vi "realtime_I_K6221_vs_time_PK.vi"() -> ()   [LabVIEW 2016]
uses:
  <instrlib>/Keithley 622x LV 2009/Utility/Typedefs/KE622x -- Instrument Type.ctl
  <instrlib>/Keithley 622x LV 2009/Keithley 622x.lvlib
panel:
  in  "Instrument Type":T1=enum."KE6221"
  in  "K6221":refnum<visa-resource-name>="GPIB0::26::INSTR"
  out "Time(s)":dbl format="%#_13g"
  out "No. of data points collected":i32
  out "Current (A)":dbl=nan
  out "Current vs time":cluster{dbl, "Field Reading":dbl}[](graph)=[{0.0, "Field Reading"=1.0754909033057532e-08}, {4.551, "Field Reading"=1.0775176727399796e-08}, {9.079, "Field Reading"=1.0695936548822218e-08}, {13.636, "Field Reading"=1.0701268908690468e-08}, {18.154, "Field Reading"=1.0658796866433243e-08}, {22.685, "Field Reading"=1.0644955615895597e-08}, {27.196, "Field Reading"=1.0609443608454975e-08}, {31.764, "Field Reading"=1.0588135917913612e-08}, {36.283, "Field Reading"=1.0537267739517534e-08}, {40.802, "Field Reading"=1.0571090092717568e-08}, {45.37, "Field Reading"=1.0597450432074013e-08}, {49.892, "Field Reading"=1.0554082828015275e-08}, {54.416, "Field Reading"=1.0529144396930967e-08}, {58.975, "Field Reading"=1.0525243011530484e-08}, {63.495, "Field Reading"=1.0496422204909802e-08}, {68.076, "Field Reading"=1.0537492386015997e-08}, {72.594, "Field Reading"=1.041855360011532e-08}, {77.111, "Field Reading"=1.0414805764361074e-08}, {81.633, "Field Reading"=1.0427666088764133e-08}, {86.192, "Field Reading"=1.040983248991928e-08}, {90.711, "Field Reading"=1.0415274184948404e-08}, {95.278, "Field Reading"=1.0351658780517077e-08}, {99.809, "Field Reading"=1.0347778042711309e-08}, {104.32, "Field Reading"=1.0404151525170418e-08}, {108.897, "Field Reading"=1.0367328564547418e-08}, {113.406, "Field Reading"=1.035592250362828e-08}, {117.929, "Field Reading"=1.034164711520283e-08}, {122.501, "Field Reading"=1.0372545079311634e-08}, {127.022, "Field Reading"=1.035853398570497e-08}, {131.534, "Field Reading"=1.0266362316389294e-08}, {136.112, "Field Reading"=1.0243831678579991e-08}, {140.623, "Field Reading"=1.0293090037428198e-08}, {145.201, "Field Reading"=1.025001076059906e-08}, {149.713, "Field Reading"=1.0220389068636026e-08}, {154.229, "Field Reading"=1.0367862293665633e-08}, {158.755, "Field Reading"=1.0208599005305017e-08}, {163.317, "Field Reading"=1.0248389252815388e-08}, {167.846, "Field Reading"=1.0199880715923942e-08}, {172.357, "Field Reading"=1.020809912913377e-08}, {176.927, "Field Reading"=1.0004231807512444e-08}, {181.447, "Field Reading"=1.0056198083741343e-08}, {186.01, "Field Reading"=1.0175625482064012e-08}, {190.532, "Field Reading"=1.01869251911497e-08}, {195.05, "Field Reading"=1.0021725360158898e-08}, {199.622, "Field Reading"=1.0012994392348114e-08}, {204.146, "Field Reading"=9.997701041555824e-09}, {208.72, "Field Reading"=1.0014654313310312e-08}, {213.225, "Field Reading"=1.0025557506602398e-08}, {217.746, "Field Reading"=1.0035240153436886e-08}, {222.264, "Field Reading"=9.984295354303873e-09}, {226.836, "Field Reading"=9.945901881505377e-09}, {231.363, "Field Reading"=9.909901055069444e-09}, {235.87, "Field Reading"=9.879079688367416e-09}, {240.45, "Field Reading"=9.871891153879234e-09}, {244.957, "Field Reading"=9.820091191293928e-09}, {249.483, "Field Reading"=9.868208637490788e-09}, {254.057, "Field Reading"=9.723922102520499e-09}, {258.569, "Field Reading"=9.810851178546986e-09}, {263.137, "Field Reading"=9.868075070608025e-09}, {267.653, "Field Reading"=9.838459710300165e-09}, {272.232, "Field Reading"=9.794170154639246e-09}, {276.743, "Field Reading"=9.8240656612309e-09}, {281.263, "Field Reading"=9.816160129037189e-09}, {285.784, "Field Reading"=9.76028149014062e-09}, {290.358, "Field Reading"=9.770277657564933e-09}, {294.874, "Field Reading"=9.746852359819687e-09}, {299.449, "Field Reading"=9.691761324726048e-09}, {303.963, "Field Reading"=9.684356029780129e-09}, {308.532, "Field Reading"=9.679807729280934e-09}, {313.057, "Field Reading"=9.640167724579342e-09}, {317.576, "Field Reading"=9.651175663070228e-09}, {322.083, "Field Reading"=9.58822823601118e-09}, {326.663, "Field Reading"=9.599135974960226e-09}, {331.185, "Field Reading"=9.598302330065866e-09}, {335.749, "Field Reading"=9.594917386794453e-09}, {340.262, "Field Reading"=9.525752610701409e-09}, {344.782, "Field Reading"=9.535515829352e-09}, {349.309, "Field Reading"=9.561137526842156e-09}, {353.874, "Field Reading"=9.584085744924857e-09}, {358.396, "Field Reading"=9.477114337135297e-09}, {362.912, "Field Reading"=9.447686796961366e-09}, {367.477, "Field Reading"=9.456034130056011e-09}, {372.052, "Field Reading"=9.553141057667689e-09}, {376.566, "Field Reading"=9.493894961055902e-09}, {381.085, "Field Reading"=9.512667690597965e-09}, {385.602, "Field Reading"=9.474293153796591e-09}, {390.171, "Field Reading"=9.48223505565176e-09}, {394.688, "Field Reading"=9.445833232680502e-09}, {399.211, "Field Reading"=9.435606847282211e-09}, {403.78, "Field Reading"=9.392508049903565e-09}, {408.307, "Field Reading"=9.449390881958631e-09}, {412.825, "Field Reading"=9.387147868215114e-09}, {417.398, "Field Reading"=9.385493712017552e-09}, {421.906, "Field Reading"=9.400358378971229e-09}, {426.424, "Field Reading"=9.398262149895849e-09}, {430.944, "Field Reading"=9.293325719135014e-09}, {435.509, "Field Reading"=9.25682735507907e-09}, {440.034, "Field Reading"=9.374365520285052e-09}, {444.553, "Field Reading"=9.318008914318868e-09}, {449.118, "Field Reading"=9.379955683639186e-09}, {453.644, "Field Reading"=9.253105241135013e-09}, {458.209, "Field Reading"=9.328575358279307e-09}, {462.734, "Field Reading"=9.253544243941528e-09}, {467.255, "Field Reading"=9.25991158545122e-09}, {471.816, "Field Reading"=9.284130103339946e-09}, {476.34, "Field Reading"=9.260943222993443e-09}, {480.855, "Field Reading"=9.221960949633347e-09}, {485.445, "Field Reading"=9.185801120431644e-09}, {489.94, "Field Reading"=9.159181944365167e-09}, {494.463, "Field Reading"=9.209935281527626e-09}, {499.034, "Field Reading"=9.19608375149852e-09}, {503.556, "Field Reading"=9.182985788676442e-09}, {508.068, "Field Reading"=9.165322100062373e-09}, {512.638, "Field Reading"=9.211178101816789e-09}, {517.158, "Field Reading"=9.180204858998693e-09}, {521.685, "Field Reading"=9.158994559236158e-09}, {526.255, "Field Reading"=9.1758963250259e-09}, {530.765, "Field Reading"=9.086634986873923e-09}, {535.28, "Field Reading"=9.099900873430183e-09}, {539.853, "Field Reading"=9.120829376096234e-09}, {544.369, "Field Reading"=9.087269332815875e-09}, {548.898, "Field Reading"=9.082007695288655e-09}, {553.458, "Field Reading"=9.214812031637344e-09}, {557.978, "Field Reading"=9.11252387708823e-09}, {562.496, "Field Reading"=9.072929736222325e-09}, {567.068, "Field Reading"=9.021043183178307e-09}, {571.584, "Field Reading"=9.03801125958304e-09}, {576.105, "Field Reading"=9.01631848737752e-09}, {580.673, "Field Reading"=9.050041364125796e-09}, {585.2, "Field Reading"=8.977713001804232e-09}, {589.721, "Field Reading"=8.99190890091733e-09}, {594.28, "Field Reading"=8.971478919836577e-09}, {598.808, "Field Reading"=9.086145460689195e-09}, {603.368, "Field Reading"=9.02352800831983e-09}, {607.894, "Field Reading"=9.006141316948349e-09}, {612.406, "Field Reading"=8.971321772943122e-09}, {616.977, "Field Reading"=8.87637227658503e-09}, {621.495, "Field Reading"=8.996522434369188e-09}, {626.065, "Field Reading"=8.950902247062842e-09}, {630.587, "Field Reading"=8.912383643615826e-09}, {635.103, "Field Reading"=8.976870354539083e-09}, {639.673, "Field Reading"=8.858923858160401e-09}, {644.201, "Field Reading"=8.8960051768792e-09}, {648.72, "Field Reading"=8.810199581584296e-09}, {653.288, "Field Reading"=8.895940941745202e-09}, {657.806, "Field Reading"=8.899913022850807e-09}, {662.319, "Field Reading"=8.916190881138338e-09}, {666.887, "Field Reading"=8.924042487696841e-09}, {671.406, "Field Reading"=8.914859635649715e-09}, {675.933, "Field Reading"=8.853835406217462e-09}, {680.445, "Field Reading"=8.878049398532991e-09}, {684.96, "Field Reading"=8.838628299924819e-09}, {689.49, "Field Reading"=8.86209668870415e-09}, {694.002, "Field Reading"=8.995111648514265e-09}, {698.574, "Field Reading"=8.83478014979106e-09}, {703.094, "Field Reading"=8.717619560190315e-09}, {707.609, "Field Reading"=8.712050013497354e-09}, {712.124, "Field Reading"=8.708502365357036e-09}, {716.696, "Field Reading"=8.691314966662255e-09}, {721.217, "Field Reading"=8.737746080764506e-09}, {725.797, "Field Reading"=8.754542348338075e-09}, {730.303, "Field Reading"=8.698996558397212e-09}, {734.829, "Field Reading"=8.662316813818218e-09}, {739.394, "Field Reading"=8.72618089388243e-09}, {743.923, "Field Reading"=8.65003501597524e-09}, {748.439, "Field Reading"=8.634100297220114e-09}, {753.005, "Field Reading"=8.554448175986506e-09}, {757.517, "Field Reading"=8.6470480768375e-09}, {762.093, "Field Reading"=8.627450424554927e-09}, {766.616, "Field Reading"=8.655609293037193e-09}, {771.123, "Field Reading"=8.598772636100515e-09}, {775.695, "Field Reading"=8.635154571490748e-09}, {780.223, "Field Reading"=8.581030273656012e-09}, {784.74, "Field Reading"=8.648572129901288e-09}, {789.303, "Field Reading"=8.48359186988437e-09}, {793.829, "Field Reading"=8.462186894095624e-09}, {798.341, "Field Reading"=8.449484053558205e-09}, {802.912, "Field Reading"=8.464375075519933e-09}, {807.429, "Field Reading"=8.455663326511537e-09}, {811.955, "Field Reading"=8.41671048218533e-09}, {816.517, "Field Reading"=8.431446164361004e-09}, {821.037, "Field Reading"=8.458593878169939e-09}, {825.565, "Field Reading"=8.382109947873128e-09}, {830.126, "Field Reading"=8.414584240973961e-09}, {834.696, "Field Reading"=8.37341874446073e-09}, {839.212, "Field Reading"=8.403786357243224e-09}, {843.736, "Field Reading"=8.362979579526923e-09}, {848.299, "Field Reading"=8.354055155446564e-09}, {852.829, "Field Reading"=8.404151200330487e-09}, {857.347, "Field Reading"=8.26643483008437e-09}, {861.908, "Field Reading"=8.31779272933137e-09}, {866.426, "Field Reading"=8.25824231153788e-09}, {870.954, "Field Reading"=8.300095307328627e-09}, {875.518, "Field Reading"=8.267619123556e-09}, {880.03, "Field Reading"=8.304257102384926e-09}, {884.555, "Field Reading"=8.278433629874611e-09}, {889.123, "Field Reading"=8.282911737453306e-09}, {893.651, "Field Reading"=8.199006980205121e-09}, {898.157, "Field Reading"=8.217817706466398e-09}, {902.726, "Field Reading"=8.208390958114655e-09}, {907.256, "Field Reading"=8.21453266773522e-09}, {911.779, "Field Reading"=8.281692496229213e-09}, {916.338, "Field Reading"=8.183209662741375e-09}, {920.858, "Field Reading"=8.180789889161302e-09}, {925.425, "Field Reading"=8.131614658850536e-09}, {929.954, "Field Reading"=8.120536466491654e-09}, {934.523, "Field Reading"=8.179753278006798e-09}, {939.041, "Field Reading"=8.150370290267414e-09}, {943.559, "Field Reading"=8.097291263741927e-09}, {948.069, "Field Reading"=8.081965073165587e-09}, {952.64, "Field Reading"=8.070216871005614e-09}, {957.157, "Field Reading"=8.078258465167693e-09}, {961.677, "Field Reading"=8.148352034763191e-09}, {966.242, "Field Reading"=8.122407244477092e-09}, {970.767, "Field Reading"=8.047340662678597e-09}, {975.293, "Field Reading"=8.002525960414962e-09}, {979.853, "Field Reading"=8.014926176603892e-09}, {984.379, "Field Reading"=7.983553304284195e-09}, {988.944, "Field Reading"=7.942024021499382e-09}, {993.46, "Field Reading"=7.970942459026299e-09}, {997.976, "Field Reading"=7.977517495385994e-09}, {1002.498, "Field Reading"=8.02506249500581e-09}, {1007.067, "Field Reading"=8.008038494822682e-09}, {1011.587, "Field Reading"=8.00819458547319e-09}, {1016.109, "Field Reading"=7.979812322773911e-09}, {1020.675, "Field Reading"=7.928940480517326e-09}, {1025.195, "Field Reading"=7.901642667764684e-09}, {1029.721, "Field Reading"=7.92334776518148e-09}, {1034.286, "Field Reading"=7.90640442487394e-09}, {1038.8, "Field Reading"=7.830530645195642e-09}, {1043.32, "Field Reading"=7.847922711437273e-09}, {1047.891, "Field Reading"=7.91455567950159e-09}, {1052.415, "Field Reading"=7.85919813738935e-09}, {1056.938, "Field Reading"=7.839264975075788e-09}, {1061.495, "Field Reading"=7.846253050845008e-09}, {1066.021, "Field Reading"=7.873822667265645e-09}, {1070.543, "Field Reading"=7.777498297266553e-09}, {1075.105, "Field Reading"=7.699228500231973e-09}, {1079.625, "Field Reading"=7.788772329837741e-09}, {1084.092, "Field Reading"=7.734988763859353e-09}, {1088.662, "Field Reading"=7.749165260772483e-09}, {1093.236, "Field Reading"=7.685132811696865e-09}, {1097.749, "Field Reading"=7.706313560812074e-09}, {1102.269, "Field Reading"=7.62077621684478e-09}, {1106.786, "Field Reading"=7.605904959160551e-09}, {1111.358, "Field Reading"=7.543054961436555e-09}, {1115.886, "Field Reading"=7.556703352397193e-09}, {1120.395, "Field Reading"=7.6113595312021e-09}, {1124.967, "Field Reading"=7.654305498550131e-09}, {1129.484, "Field Reading"=7.51327653000943e-09}, {1134.052, "Field Reading"=7.554675006342064e-09}, {1138.57, "Field Reading"=7.542420362869713e-09}, {1143.093, "Field Reading"=7.521642404769412e-09}, {1147.663, "Field Reading"=7.493718920949625e-09}, {1152.182, "Field Reading"=7.545902086235947e-09}, {1156.709, "Field Reading"=7.454572401629019e-09}, {1161.273, "Field Reading"=7.56241871334473e-09}, {1165.789, "Field Reading"=7.526457094182698e-09}, {1170.305, "Field Reading"=7.522706318451702e-09}, {1174.884, "Field Reading"=7.534649878150238e-09}, {1179.403, "Field Reading"=7.428586013070126e-09}, {1183.913, "Field Reading"=7.484029379477739e-09}, {1188.49, "Field Reading"=7.4343920904789905e-09}, {1193.011, "Field Reading"=7.431290893454047e-09}, {1197.52, "Field Reading"=7.414935186546212e-09}, {1202.092, "Field Reading"=7.46748803575265e-09}, {1206.622, "Field Reading"=7.437207307538754e-09}, {1211.176, "Field Reading"=7.378208443361683e-09}, {1215.699, "Field Reading"=7.390611615459943e-09}, {1220.216, "Field Reading"=7.388160142936117e-09}, {1224.794, "Field Reading"=7.328947288383786e-09}, {1229.304, "Field Reading"=7.319317094031018e-09}, {1233.885, "Field Reading"=7.475098348867376e-09}, {1238.392, "Field Reading"=7.530881047513595e-09}, {1242.92, "Field Reading"=7.441607140689224e-09}, {1247.441, "Field Reading"=7.46964306213466e-09}, {1252.001, "Field Reading"=7.520725885122206e-09}, {1256.518, "Field Reading"=7.492361055018034e-09}, {1261.097, "Field Reading"=7.45543070330775e-09}, {1265.608, "Field Reading"=7.555711147417944e-09}, {1270.132, "Field Reading"=7.512860653466764e-09}, {1274.695, "Field Reading"=7.400374180522194e-09}, {1279.222, "Field Reading"=7.480181197096508e-09}, {1283.732, "Field Reading"=7.49128480869075e-09}, {1288.309, "Field Reading"=7.447762196020056e-09}, {1292.823, "Field Reading"=7.534477762535263e-09}, {1297.34, "Field Reading"=7.421045122389159e-09}, {1301.915, "Field Reading"=7.440020494736612e-09}, {1306.431, "Field Reading"=7.390355809789666e-09}, {1310.947, "Field Reading"=7.455811921741306e-09}, {1315.469, "Field Reading"=7.344696388910505e-09}, {1320.038, "Field Reading"=7.361054012595228e-09}, {1324.554, "Field Reading"=7.379124594102075e-09}, {1329.125, "Field Reading"=7.224554592996079e-09}, {1333.643, "Field Reading"=7.260924217923489e-09}, {1338.221, "Field Reading"=7.2892639063543325e-09}, {1342.731, "Field Reading"=7.315390774955184e-09}, {1347.261, "Field Reading"=7.248524038949682e-09}, {1351.772, "Field Reading"=7.325095750213407e-09}, {1356.337, "Field Reading"=7.336315701547141e-09}, {1360.865, "Field Reading"=7.278166100536928e-09}, {1365.377, "Field Reading"=7.163994031886997e-09}, {1369.958, "Field Reading"=7.27625701148584e-09}, {1374.476, "Field Reading"=7.222396143186761e-09}, {1378.996, "Field Reading"=7.1660041850257785e-09}, {1383.561, "Field Reading"=7.206045462597249e-09}, {1388.072, "Field Reading"=7.128329621712486e-09}, {1392.651, "Field Reading"=7.056225847998549e-09}, {1397.158, "Field Reading"=7.11894838847704e-09}, {1401.689, "Field Reading"=6.983910482704493e-09}, {1406.25, "Field Reading"=7.125065175778337e-09}, {1410.769, "Field Reading"=7.0718729037374506e-09}, {1415.288, "Field Reading"=7.066078412703073e-09}, {1419.865, "Field Reading"=7.1240268833397976e-09}, {1424.376, "Field Reading"=7.090289281222082e-09}, {1428.895, "Field Reading"=7.079182013812105e-09}, {1433.466, "Field Reading"=7.052866686174349e-09}, {1437.984, "Field Reading"=7.008290615374676e-09}, {1442.561, "Field Reading"=7.010020496732931e-09}, {1447.077, "Field Reading"=6.989410914801963e-09}, {1451.597, "Field Reading"=7.034265387395938e-09}, {1456.168, "Field Reading"=6.9810102143820956e-09}, {1460.677, "Field Reading"=6.938299286302394e-09}, {1465.197, "Field Reading"=6.978178942042398e-09}, {1469.727, "Field Reading"=6.8779042070236515e-09}, {1474.295, "Field Reading"=6.941235031485825e-09}, {1478.806, "Field Reading"=6.974993006879735e-09}, {1483.374, "Field Reading"=6.9304914236992475e-09}, {1487.893, "Field Reading"=6.914604243080792e-09}, {1492.411, "Field Reading"=6.8790622070962475e-09}, {1496.988, "Field Reading"=6.932513993349057e-09}, {1501.5, "Field Reading"=6.85674880566968e-09}, {1506.032, "Field Reading"=6.8528700192297855e-09}, {1510.597, "Field Reading"=6.808052132425589e-09}, {1515.108, "Field Reading"=6.835183113829124e-09}, {1519.678, "Field Reading"=6.843735327128739e-09}, {1524.205, "Field Reading"=6.82318085777842e-09}, {1528.724, "Field Reading"=6.832044008852625e-09}, {1533.286, "Field Reading"=6.802117140648846e-09}, {1537.803, "Field Reading"=6.772844086155588e-09}, {1542.323, "Field Reading"=6.822945389946027e-09}, {1546.904, "Field Reading"=6.839929552184977e-09}, {1551.414, "Field Reading"=6.760385900681559e-09}, {1555.926, "Field Reading"=6.778053378494218e-09}, {1560.497, "Field Reading"=6.703948346977387e-09}, {1565.015, "Field Reading"=6.563250547926023e-09}, {1569.543, "Field Reading"=6.6299234131757845e-09}, {1574.104, "Field Reading"=6.736966390143081e-09}, {1578.625, "Field Reading"=6.679466270417032e-09}, {1583.146, "Field Reading"=6.7137766003536715e-09}, {1587.712, "Field Reading"=6.7748645552631824e-09}, {1592.238, "Field Reading"=6.719927412700429e-09}, {1596.811, "Field Reading"=6.730824453621419e-09}, {1601.329, "Field Reading"=6.663369976605285e-09}, {1605.84, "Field Reading"=6.707049341481758e-09}, {1610.408, "Field Reading"=6.684630551707419e-09}, {1614.938, "Field Reading"=6.664691616251728e-09}, {1619.453, "Field Reading"=6.656185262646725e-09}, {1624.013, "Field Reading"=6.6765590388699805e-09}, {1628.534, "Field Reading"=6.62265260165533e-09}, {1633.053, "Field Reading"=6.674574864862748e-09}, {1637.625, "Field Reading"=6.675736004747752e-09}, {1642.142, "Field Reading"=6.60537085887356e-09}, {1646.66, "Field Reading"=6.6637996325844384e-09}, {1651.228, "Field Reading"=6.5961502972892314e-09}, {1655.749, "Field Reading"=6.596303887361527e-09}, {1660.274, "Field Reading"=6.571446866486034e-09}, {1664.847, "Field Reading"=6.529502602168678e-09}, {1669.354, "Field Reading"=6.527421029407293e-09}, {1673.885, "Field Reading"=6.540766029865476e-09}, {1678.451, "Field Reading"=6.492829708078334e-09}, {1682.965, "Field Reading"=6.4955920158181225e-09}, {1687.493, "Field Reading"=6.524742446336385e-09}, {1692.064, "Field Reading"=6.531316113124561e-09}, {1696.573, "Field Reading"=6.4567670106243025e-09}, {1701.088, "Field Reading"=6.5145716741219224e-09}, {1705.666, "Field Reading"=6.437718489025235e-09}, {1710.176, "Field Reading"=6.434858544194384e-09}, {1714.705, "Field Reading"=6.421443345821634e-09}, {1719.269, "Field Reading"=6.371481839753699e-09}, {1723.788, "Field Reading"=6.296068293356122e-09}, {1728.306, "Field Reading"=6.35027174500087e-09}, {1732.875, "Field Reading"=6.454036642676171e-09}, {1737.401, "Field Reading"=6.380828265542994e-09}, {1741.913, "Field Reading"=6.34284100311131e-09}, {1746.48, "Field Reading"=6.388160792710688e-09}, {1751.01, "Field Reading"=6.325737961738322e-09}, {1755.526, "Field Reading"=6.342308453232134e-09}, {1760.037, "Field Reading"=6.333324326492032e-09}, {1764.604, "Field Reading"=6.384382451809395e-09}, {1769.175, "Field Reading"=6.2830842660487484e-09}, {1773.653, "Field Reading"=6.329756591029826e-09}, {1778.211, "Field Reading"=6.287710307125148e-09}, {1782.735, "Field Reading"=6.23671601406328e-09}, {1787.3, "Field Reading"=6.2104120139809386e-09}, {1791.829, "Field Reading"=6.248345131813233e-09}, {1796.337, "Field Reading"=6.203355760520761e-09}, {1800.92, "Field Reading"=6.245820454192768e-09}, {1805.429, "Field Reading"=6.2299160758381866e-09}, {1810.001, "Field Reading"=6.2198009398469865e-09}, {1814.517, "Field Reading"=6.179484780405028e-09}, {1819.033, "Field Reading"=6.1599705063695305e-09}, {1823.613, "Field Reading"=6.115058689956539e-09}, {1828.134, "Field Reading"=6.14494700018927e-09}, {1832.652, "Field Reading"=6.119665888529578e-09}, {1837.223, "Field Reading"=6.0734460460054165e-09}, {1841.734, "Field Reading"=6.098860598174129e-09}, {1846.249, "Field Reading"=6.0892519425498796e-09}, {1850.822, "Field Reading"=6.0633158371077235e-09}, {1855.347, "Field Reading"=5.948363297347473e-09}, {1859.859, "Field Reading"=6.0406330176099355e-09}, {1864.427, "Field Reading"=6.004073124008287e-09}, {1868.957, "Field Reading"=6.029851836007183e-09}, {1873.473, "Field Reading"=5.9914187753561554e-09}, {1878.034, "Field Reading"=5.999767415441637e-09}, {1882.552, "Field Reading"=6.117321346379777e-09}, {1887.08, "Field Reading"=5.984033037553823e-09}, {1891.647, "Field Reading"=5.982285937087253e-09}, {1896.159, "Field Reading"=5.990168025933193e-09}, {1900.689, "Field Reading"=6.004257979431128e-09}, {1905.248, "Field Reading"=5.988751466153552e-09}, {1909.767, "Field Reading"=5.952918589405235e-09}, {1914.286, "Field Reading"=5.9346022587389726e-09}, {1918.854, "Field Reading"=6.06224562335777e-09}, {1923.374, "Field Reading"=5.9882646744531435e-09}, {1927.904, "Field Reading"=5.910311645124628e-09}, {1932.474, "Field Reading"=5.907578635180826e-09}, {1936.981, "Field Reading"=5.809968219029195e-09}, {1941.511, "Field Reading"=5.8937340716148185e-09}, {1946.08, "Field Reading"=5.857486959453094e-09}, {1950.59, "Field Reading"=5.8921225060025876e-09}, {1955.109, "Field Reading"=5.843412764586583e-09}, {1959.686, "Field Reading"=5.840361982828319e-09}, {1964.198, "Field Reading"=5.876345012916096e-09}, {1968.726, "Field Reading"=5.6424857524202175e-09}, {1973.296, "Field Reading"=5.584454321472799e-09}, {1977.805, "Field Reading"=5.518517462180017e-09}, {1982.319, "Field Reading"=5.492298065847143e-09}, {1986.892, "Field Reading"=5.556064858887497e-09}, {1991.421, "Field Reading"=5.511080763648863e-09}, {1995.93, "Field Reading"=5.5534959767069855e-09}, {2000.507, "Field Reading"=5.390655559323085e-09}, {2005.017, "Field Reading"=5.5196174128002705e-09}, {2009.546, "Field Reading"=5.524330397641961e-09}, {2014.114, "Field Reading"=5.551279674473231e-09}, {2018.636, "Field Reading"=5.441456111231054e-09}, {2023.144, "Field Reading"=5.511133359960133e-09}, {2027.715, "Field Reading"=5.508735345064296e-09}, {2032.242, "Field Reading"=5.464306100812849e-09}, {2036.805, "Field Reading"=5.4387948009573845e-09}, {2041.328, "Field Reading"=5.412199127600727e-09}, {2045.841, "Field Reading"=5.403678836423456e-09}, {2050.366, "Field Reading"=5.408782038343089e-09}, {2054.938, "Field Reading"=5.3732110038646596e-09}, {2059.448, "Field Reading"=5.419766380383462e-09}, {2063.968, "Field Reading"=5.376757868673863e-09}, {2068.544, "Field Reading"=5.3396410130995e-09}, {2073.068, "Field Reading"=5.36724469983585e-09}, {2077.584, "Field Reading"=5.3735942125553935e-09}, {2082.143, "Field Reading"=5.3468592999880246e-09}, {2086.663, "Field Reading"=5.3010485259838155e-09}, {2091.187, "Field Reading"=5.456036409406565e-09}, {2095.762, "Field Reading"=5.280868790779229e-09}, {2100.27, "Field Reading"=5.286862768294893e-09}, {2104.789, "Field Reading"=5.247716712141317e-09}, {2109.315, "Field Reading"=5.278849454886213e-09}, {2113.825, "Field Reading"=5.2923297743841376e-09}, {2118.395, "Field Reading"=5.270920000524356e-09}, {2122.923, "Field Reading"=5.2426548936782815e-09}, {2127.433, "Field Reading"=5.280403805069135e-09}, {2132.005, "Field Reading"=5.2319073098520134e-09}, {2136.519, "Field Reading"=5.231685501327516e-09}, {2141.044, "Field Reading"=5.259824922125597e-09}, {2145.568, "Field Reading"=5.247182807747317e-09}, {2150.128, "Field Reading"=5.190062070131187e-09}, {2154.648, "Field Reading"=5.184434911997065e-09}, {2159.217, "Field Reading"=5.188293654611709e-09}, {2163.737, "Field Reading"=5.1899556848997125e-09}, {2168.266, "Field Reading"=5.0888494780519e-09}, {2172.832, "Field Reading"=5.248582300166497e-09}, {2177.35, "Field Reading"=5.076499164263517e-09}, {2181.863, "Field Reading"=5.131572283172578e-09}, {2186.442, "Field Reading"=5.125631012119856e-09}, {2190.952, "Field Reading"=4.9843218111128326e-09}, {2195.47, "Field Reading"=4.9996711481800855e-09}, {2200.0, "Field Reading"=5.101682906041411e-09}, {2204.567, "Field Reading"=5.1194617917379804e-09}, {2209.08, "Field Reading"=5.083836655011101e-09}, {2213.646, "Field Reading"=5.171637385896983e-09}, {2218.175, "Field Reading"=5.071765268012458e-09}, {2222.683, "Field Reading"=5.099376175962705e-09}, {2227.261, "Field Reading"=5.234327770348536e-09}, {2231.781, "Field Reading"=5.051878025946999e-09}, {2236.29, "Field Reading"=5.049711877490007e-09}, {2240.871, "Field Reading"=5.075759925283179e-09}, {2245.385, "Field Reading"=5.049338460575e-09}, {2249.903, "Field Reading"=5.0161356893027244e-09}, {2254.427, "Field Reading"=5.0230183241736195e-09}, {2258.988, "Field Reading"=5.030438687173533e-09}, {2263.514, "Field Reading"=4.994739674182154e-09}, {2268.08, "Field Reading"=4.9525300147223835e-09}, {2272.594, "Field Reading"=4.963937554569273e-09}, {2277.117, "Field Reading"=5.045702938207714e-09}, {2281.641, "Field Reading"=5.06722918172536e-09}, {2286.202, "Field Reading"=4.973308396162686e-09}, {2290.722, "Field Reading"=4.9236264336615236e-09}, {2295.297, "Field Reading"=4.916131301155814e-09}, {2299.812, "Field Reading"=4.714144468453278e-09}, {2304.337, "Field Reading"=4.8578439153711055e-09}, {2308.901, "Field Reading"=4.944636774131635e-09}, {2313.424, "Field Reading"=4.915460953881695e-09}, {2317.936, "Field Reading"=4.9040316230072865e-09}, {2322.509, "Field Reading"=4.935556907548174e-09}, {2327.039, "Field Reading"=4.693195742340591e-09}, {2331.549, "Field Reading"=4.8365933169312125e-09}, {2336.112, "Field Reading"=4.873741611898118e-09}, {2340.627, "Field Reading"=4.87098306879858e-09}, {2345.149, "Field Reading"=4.886643394918473e-09}, {2349.731, "Field Reading"=4.847161699026444e-09}, {2354.241, "Field Reading"=4.8095999601051754e-09}, {2358.769, "Field Reading"=4.853600025776515e-09}, {2363.327, "Field Reading"=4.799468080468557e-09}, {2367.847, "Field Reading"=4.7953475602903006e-09}, {2372.418, "Field Reading"=4.793214078216478e-09}, {2376.933, "Field Reading"=4.810840226103454e-09}, {2381.454, "Field Reading"=4.865078341668466e-09}, {2385.977, "Field Reading"=4.840969885706196e-09}, {2390.542, "Field Reading"=4.795338710939571e-09}, {2395.073, "Field Reading"=4.764189348002715e-09}, {2399.63, "Field Reading"=4.830336643018953e-09}, {2404.149, "Field Reading"=4.767794564180055e-09}, {2408.669, "Field Reading"=4.759573115020579e-09}, {2413.24, "Field Reading"=4.733653930103231e-09}, {2417.756, "Field Reading"=4.7333887318652545e-09}, {2422.276, "Field Reading"=4.756180784291175e-09}, {2426.795, "Field Reading"=4.726306449651303e-09}, {2431.312, "Field Reading"=4.754839532191907e-09}, {2435.835, "Field Reading"=4.7155584472565435e-09}, {2440.41, "Field Reading"=4.73226902156852e-09}, {2444.93, "Field Reading"=4.702601943098045e-09}, {2449.486, "Field Reading"=4.690999622204039e-09}, {2454.012, "Field Reading"=4.704904091220417e-09}, {2458.539, "Field Reading"=4.720155874749969e-09}, {2463.097, "Field Reading"=4.696692483453088e-09}, {2467.617, "Field Reading"=4.750636089388704e-09}, {2472.136, "Field Reading"=4.6349266909897594e-09}, {2476.709, "Field Reading"=4.616489831374194e-09}, {2481.233, "Field Reading"=4.653917179284386e-09}, {2485.743, "Field Reading"=4.597179099237373e-09}, {2490.322, "Field Reading"=4.62965768290453e-09}, {2494.843, "Field Reading"=4.580876998137564e-09}, {2499.35, "Field Reading"=4.563605566215481e-09}, {2503.929, "Field Reading"=4.482156621094803e-09}, {2508.438, "Field Reading"=4.56564412586279e-09}, {2512.967, "Field Reading"=4.6284039028636495e-09}, {2517.527, "Field Reading"=4.555885718272783e-09}, {2522.043, "Field Reading"=4.612825004734929e-09}, {2526.563, "Field Reading"=4.562173111447981e-09}, {2531.133, "Field Reading"=4.537190949114002e-09}, {2535.653, "Field Reading"=4.458793093248631e-09}, {2540.173, "Field Reading"=4.52847678054535e-09}, {2544.751, "Field Reading"=4.5208203520489556e-09}, {2549.261, "Field Reading"=4.488778286223336e-09}, {2553.836, "Field Reading"=4.515060848155167e-09}, {2558.346, "Field Reading"=4.535677882101488e-09}, {2562.865, "Field Reading"=4.491433730517111e-09}, {2567.446, "Field Reading"=4.40054650332015e-09}, {2571.958, "Field Reading"=4.4486768815728506e-09}, {2576.479, "Field Reading"=4.450401351523994e-09}, {2581.045, "Field Reading"=4.487487042996042e-09}, {2585.57, "Field Reading"=4.521073558541402e-09}, {2590.087, "Field Reading"=4.480317491831756e-09}, {2594.66, "Field Reading"=4.447220429955687e-09}, {2599.173, "Field Reading"=4.465278706563569e-09}, {2603.689, "Field Reading"=4.530833160445025e-09}, {2608.256, "Field Reading"=4.46058555065712e-09}, {2612.78, "Field Reading"=4.5023304179226495e-09}, {2617.303, "Field Reading"=4.4984738593324374e-09}, {2621.873, "Field Reading"=4.464385171352175e-09}, {2626.392, "Field Reading"=4.420344688673969e-09}, {2630.903, "Field Reading"=4.4605510979104775e-09}, {2635.473, "Field Reading"=4.456349305462267e-09}, {2639.992, "Field Reading"=4.447282413922074e-09}, {2644.521, "Field Reading"=4.4005362081489584e-09}, {2649.084, "Field Reading"=4.419815677897478e-09}, {2653.599, "Field Reading"=4.4490627238802725e-09}, {2658.12, "Field Reading"=4.426216132762487e-09}, {2662.698, "Field Reading"=4.438934041368195e-09}, {2667.205, "Field Reading"=4.387900945403299e-09}, {2671.774, "Field Reading"=4.382516342217813e-09}, {2676.292, "Field Reading"=4.305606998657238e-09}, {2680.822, "Field Reading"=4.294156755498741e-09}, {2685.334, "Field Reading"=4.325699346091874e-09}, {2689.904, "Field Reading"=4.350499875913346e-09}, {2694.421, "Field Reading"=4.311755905277652e-09}, {2699.002, "Field Reading"=4.363645908173991e-09}, {2703.51, "Field Reading"=4.1120668202905374e-09}, {2708.028, "Field Reading"=4.295205176022663e-09}, {2712.608, "Field Reading"=4.36896282308688e-09}, {2717.116, "Field Reading"=4.321470983999847e-09}, {2721.638, "Field Reading"=4.302651668919814e-09}, {2726.156, "Field Reading"=4.343242620484273e-09}, {2730.683, "Field Reading"=4.323224041888555e-09}, {2735.193, "Field Reading"=4.310553141307406e-09}, {2739.764, "Field Reading"=4.287275008586955e-09}, {2744.289, "Field Reading"=4.3036975096247464e-09}, {2748.81, "Field Reading"=4.28300162428243e-09}, {2753.369, "Field Reading"=4.256592486673957e-09}, {2757.887, "Field Reading"=4.280138631155222e-09}, {2762.466, "Field Reading"=4.273882262990543e-09}, {2766.979, "Field Reading"=4.245510304975803e-09}, {2771.499, "Field Reading"=4.2518408662365565e-09}, {2776.071, "Field Reading"=4.257914238376479e-09}, {2780.594, "Field Reading"=4.275778982939147e-09}, {2785.102, "Field Reading"=4.274537782607576e-09}, {2789.682, "Field Reading"=4.257539260653195e-09}, {2794.189, "Field Reading"=4.281552810888528e-09}, {2798.719, "Field Reading"=4.272569423208378e-09}, {2803.282, "Field Reading"=4.2507998521794185e-09}, {2807.806, "Field Reading"=4.402992020617553e-09}, {2812.379, "Field Reading"=4.333066717448041e-09}, {2816.889, "Field Reading"=4.1775869387219764e-09}, {2821.406, "Field Reading"=4.206061747441249e-09}, {2825.925, "Field Reading"=4.229249997577112e-09}, {2830.502, "Field Reading"=4.199507996530501e-09}, {2835.01, "Field Reading"=4.2149095193546955e-09}, {2839.583, "Field Reading"=4.1620925752143e-09}, {2844.112, "Field Reading"=4.157359913307775e-09}, {2848.63, "Field Reading"=4.235946556959495e-09}, {2853.2, "Field Reading"=4.260280168856574e-09}, {2857.707, "Field Reading"=4.242102000418811e-09}, {2862.226, "Field Reading"=4.221770054542564e-09}, {2866.797, "Field Reading"=4.155441673510657e-09}, {2871.313, "Field Reading"=4.12733803293591e-09}, {2875.884, "Field Reading"=4.098412378179983e-09}, {2880.403, "Field Reading"=4.099452088432523e-09}, {2884.919, "Field Reading"=4.1155581045556815e-09}, {2889.499, "Field Reading"=4.135260309733198e-09}, {2894.022, "Field Reading"=4.114071010222697e-09}, {2898.532, "Field Reading"=4.069242642699316e-09}, {2903.11, "Field Reading"=4.097304638802798e-09}, {2907.617, "Field Reading"=4.133325263525135e-09}, {2912.147, "Field Reading"=4.0964011984037445e-09}, {2916.718, "Field Reading"=4.076996941143137e-09}, {2921.236, "Field Reading"=4.089355976700678e-09}, {2925.754, "Field Reading"=4.132212860708971e-09}, {2930.323, "Field Reading"=4.0736267591976685e-09}, {2934.835, "Field Reading"=4.078643953597773e-09}, {2939.349, "Field Reading"=4.012473284259884e-09}, {2943.929, "Field Reading"=4.036056995358176e-09}, {2948.445, "Field Reading"=4.077616232464626e-09}, {2952.968, "Field Reading"=4.029426057819201e-09}, {2957.525, "Field Reading"=4.230247682223658e-09}, {2962.047, "Field Reading"=4.033582972882056e-09}, {2966.576, "Field Reading"=4.017768348363297e-09}, {2971.137, "Field Reading"=4.035847466348764e-09}, {2975.655, "Field Reading"=3.998299780088036e-09}, {2980.171, "Field Reading"=3.990711972264081e-09}, {2984.742, "Field Reading"=3.964267980481467e-09}, {2989.274, "Field Reading"=3.967521997494993e-09}, {2993.83, "Field Reading"=4.018937217699934e-09}, {2998.351, "Field Reading"=4.027985733896478e-09}, {3002.87, "Field Reading"=3.997779074644891e-09}, {3007.391, "Field Reading"=3.97031698501138e-09}, {3011.957, "Field Reading"=3.97039487982801e-09}, {3016.48, "Field Reading"=3.979889807500979e-09}, {3021.056, "Field Reading"=3.9984174608503344e-09}, {3025.571, "Field Reading"=3.983326985431952e-09}, {3030.083, "Field Reading"=3.953506001521022e-09}, {3034.66, "Field Reading"=3.967967411850339e-09}, {3039.174, "Field Reading"=3.949281177625683e-09}, {3043.695, "Field Reading"=3.925378907646012e-09}, {3048.261, "Field Reading"=3.926174603156441e-09}, {3052.788, "Field Reading"=3.9055722230863814e-09}, {3057.309, "Field Reading"=3.892840735178282e-09}, {3061.814, "Field Reading"=3.889667787686983e-09}, {3066.388, "Field Reading"=3.941366575079191e-09}, {3070.914, "Field Reading"=3.895250093627123e-09}, {3075.438, "Field Reading"=3.93016989438934e-09}, {3079.991, "Field Reading"=3.889595124568379e-09}, {3084.519, "Field Reading"=3.897620337295719e-09}, {3089.082, "Field Reading"=3.9288425604617075e-09}, {3093.601, "Field Reading"=3.916354345820998e-09}, {3098.121, "Field Reading"=3.8659781503571734e-09}, {3102.691, "Field Reading"=3.891155109635458e-09}, {3107.209, "Field Reading"=3.880666096033378e-09}, {3111.787, "Field Reading"=3.84664344310953e-09}, {3116.305, "Field Reading"=3.881536845936245e-09}, {3120.817, "Field Reading"=3.829417679779926e-09}, {3125.388, "Field Reading"=3.811574465176615e-09}, {3129.91, "Field Reading"=3.804852423751292e-09}, {3134.436, "Field Reading"=3.874432111391402e-09}, {3138.954, "Field Reading"=3.86923808460875e-09}, {3143.518, "Field Reading"=3.873514424891525e-09}, {3148.039, "Field Reading"=3.8954065143834715e-09}, {3152.609, "Field Reading"=3.9153415981751845e-09}, {3157.127, "Field Reading"=3.877234052295817e-09}, {3161.635, "Field Reading"=3.8638428965216884e-09}, {3166.163, "Field Reading"=3.849535446893198e-09}, {3170.726, "Field Reading"=3.870498790296755e-09}, {3175.246, "Field Reading"=3.961301168922662e-09}, {3179.81, "Field Reading"=3.82901202506132e-09}, {3184.334, "Field Reading"=3.855100134606814e-09}, {3188.851, "Field Reading"=3.866319303247789e-09}, {3193.419, "Field Reading"=3.829821600240689e-09}, {3197.948, "Field Reading"=3.888143158979643e-09}, {3202.458, "Field Reading"=3.857915449375062e-09}, {3207.034, "Field Reading"=3.901901346986651e-09}, {3211.546, "Field Reading"=3.957888493146684e-09}, {3216.065, "Field Reading"=3.828920529354855e-09}, {3220.634, "Field Reading"=3.795590786762854e-09}, {3225.155, "Field Reading"=3.800565934073015e-09}, {3229.681, "Field Reading"=3.928171499560289e-09}, {3234.24, "Field Reading"=3.786240229699521e-09}, {3238.767, "Field Reading"=3.793366454230641e-09}, {3243.284, "Field Reading"=3.8521504698029135e-09}, {3247.861, "Field Reading"=3.845378204133779e-09}, {3252.379, "Field Reading"=3.8030659298234855e-09}, {3256.895, "Field Reading"=3.80822870404292e-09}, {3261.459, "Field Reading"=3.853876555590036e-09}, {3265.977, "Field Reading"=3.838449438576926e-09}, {3270.503, "Field Reading"=3.800306369891086e-09}, {3275.069, "Field Reading"=3.812232283001766e-09}, {3279.587, "Field Reading"=3.80105672796973e-09}, {3284.166, "Field Reading"=3.941290676552618e-09}, {3288.671, "Field Reading"=3.7600473908784135e-09}, {3293.195, "Field Reading"=3.829816077357103e-09}, {3297.763, "Field Reading"=3.8099605136580064e-09}, {3302.283, "Field Reading"=3.767741358846101e-09}, {3306.807, "Field Reading"=3.731807126710847e-09}, {3311.369, "Field Reading"=3.7328483734789136e-09}, {3315.886, "Field Reading"=3.754624255671522e-09}, {3320.407, "Field Reading"=3.756348928240287e-09}, {3324.977, "Field Reading"=3.7676809607753496e-09}, {3329.498, "Field Reading"=3.734718682627865e-09}, {3334.024, "Field Reading"=3.7290158336426605e-09}, {3338.583, "Field Reading"=3.6633639770500477e-09}, {3343.104, "Field Reading"=3.7091299984409564e-09}, {3347.672, "Field Reading"=3.702057361509842e-09}, {3352.199, "Field Reading"=3.752512697421581e-09}, {3356.718, "Field Reading"=3.751191129059365e-09}, {3361.287, "Field Reading"=3.7276886913583535e-09}, {3365.798, "Field Reading"=3.708359096372794e-09}, {3370.319, "Field Reading"=3.6572451680989307e-09}, {3374.885, "Field Reading"=3.654821316365914e-09}, {3379.413, "Field Reading"=3.661360105795853e-09}, {3383.932, "Field Reading"=3.702827717783641e-09}, {3388.501, "Field Reading"=3.6915953198026196e-09}, {3393.023, "Field Reading"=3.6650692034509655e-09}, {3397.534, "Field Reading"=3.7183524095892414e-09}, {3402.1, "Field Reading"=3.6606869532280256e-09}, {3406.619, "Field Reading"=3.6923454877441593e-09}, {3411.138, "Field Reading"=3.7045651779042562e-09}, {3415.716, "Field Reading"=3.722736172894848e-09}, {3420.226, "Field Reading"=3.6686444683682193e-09}, {3424.751, "Field Reading"=3.6617341221891195e-09}, {3429.274, "Field Reading"=3.6624672160304364e-09}, {3433.835, "Field Reading"=3.6706625418622536e-09}, {3438.401, "Field Reading"=3.657853174941169e-09}, {3442.923, "Field Reading"=3.631895438387292e-09}, {3447.451, "Field Reading"=3.602604002921477e-09}, {3452.013, "Field Reading"=3.653414577476343e-09}, {3456.528, "Field Reading"=3.5248826111565364e-09}, {3461.049, "Field Reading"=3.628658013142907e-09}, {3465.618, "Field Reading"=3.6301541943119703e-09}, {3470.143, "Field Reading"=3.6020370859448597e-09}, {3474.658, "Field Reading"=3.617553063600344e-09}, {3479.181, "Field Reading"=3.5738443070048718e-09}, {3483.743, "Field Reading"=3.574076843211482e-09}, {3488.266, "Field Reading"=3.5955945411022413e-09}, {3492.78, "Field Reading"=3.5820984349559713e-09}, {3497.352, "Field Reading"=3.581313038529724e-09}, {3501.879, "Field Reading"=3.553751533228934e-09}, {3506.396, "Field Reading"=3.5651475752506964e-09}, {3510.968, "Field Reading"=3.5849016057066314e-09}, {3515.476, "Field Reading"=3.6260827695690775e-09}, {3520.0, "Field Reading"=3.6185048115682405e-09}, {3524.522, "Field Reading"=3.5498093093005007e-09}, {3529.096, "Field Reading"=3.5897916225569617e-09}, {3533.603, "Field Reading"=3.5568948002622894e-09}, {3538.122, "Field Reading"=3.546624575003056e-09}, {3542.692, "Field Reading"=3.5427213892132645e-09}, {3547.211, "Field Reading"=3.594172348880362e-09}, {3551.786, "Field Reading"=3.587896179631731e-09}, {3556.306, "Field Reading"=3.5302965486685286e-09}, {3560.828, "Field Reading"=3.5274422683042437e-09}, {3565.336, "Field Reading"=3.5455849170809744e-09}, {3569.916, "Field Reading"=3.548000808028428e-09}, {3574.429, "Field Reading"=3.504485089136315e-09}, {3578.995, "Field Reading"=3.577806240135082e-09}, {3583.514, "Field Reading"=3.5022950784820233e-09}, {3588.034, "Field Reading"=3.5653135365812712e-09}, {3592.605, "Field Reading"=3.521811013569386e-09}, {3597.122, "Field Reading"=3.5000533313086807e-09}, {3601.651, "Field Reading"=3.525407194383401e-09}, {3606.22, "Field Reading"=3.499273112744662e-09}, {3610.726, "Field Reading"=3.54045537309005e-09}, {3615.307, "Field Reading"=3.497171849058038e-09}, {3619.818, "Field Reading"=3.4504319404747347e-09}, {3624.338, "Field Reading"=3.4894412693034068e-09}, {3628.861, "Field Reading"=3.508078765650157e-09}, {3633.432, "Field Reading"=3.4918455933847735e-09}, {3637.942, "Field Reading"=3.479450262903477e-09}, {3642.523, "Field Reading"=3.444272032401606e-09}, {3647.033, "Field Reading"=3.454015315356747e-09}, {3651.549, "Field Reading"=3.447406144043503e-09}, {3656.081, "Field Reading"=3.4899293462534487e-09}, {3660.636, "Field Reading"=3.501923034361546e-09}, {3665.167, "Field Reading"=3.4856104162117454e-09}, {3669.736, "Field Reading"=3.4463248881645824e-09}, {3674.254, "Field Reading"=3.449808232151651e-09}, {3678.773, "Field Reading"=3.419809439160412e-09}, {3683.332, "Field Reading"=3.474394851377375e-09}, {3687.854, "Field Reading"=3.447175733702756e-09}, {3692.371, "Field Reading"=3.4619703714793095e-09}, {3696.944, "Field Reading"=3.4415453602652855e-09}, {3701.456, "Field Reading"=3.4070500882579844e-09}, {3705.98, "Field Reading"=3.4041063396003493e-09}, {3710.557, "Field Reading"=3.6379499472074356e-09}, {3715.081, "Field Reading"=3.4504340438868368e-09}, {3719.594, "Field Reading"=3.391965413142847e-09}, {3724.155, "Field Reading"=3.4078457011733994e-09}, {3728.679, "Field Reading"=3.4182786116738555e-09}, {3733.246, "Field Reading"=3.4890101335280267e-09}, {3737.763, "Field Reading"=3.454709663648958e-09}, {3742.29, "Field Reading"=3.4466420353281575e-09}, {3746.852, "Field Reading"=3.415634254236932e-09}, {3751.381, "Field Reading"=3.4155379895438673e-09}, {3755.887, "Field Reading"=3.362922042777208e-09}, {3760.411, "Field Reading"=3.401020275403512e-09}, {3764.978, "Field Reading"=3.399930217842445e-09}, {3769.508, "Field Reading"=3.3787086561468525e-09}, {3774.078, "Field Reading"=3.3681257595555093e-09}, {3778.594, "Field Reading"=3.390553342344768e-09}, {3783.112, "Field Reading"=3.3639937822899825e-09}, {3787.676, "Field Reading"=3.4130051871040132e-09}, {3792.193, "Field Reading"=3.4119363189705963e-09}, {3796.711, "Field Reading"=3.3697996184678692e-09}, {3801.28, "Field Reading"=3.4021238349806093e-09}, {3805.799, "Field Reading"=3.4043712703537806e-09}, {3810.318, "Field Reading"=3.383427211254074e-09}, {3814.895, "Field Reading"=3.3922213215772835e-09}, {3819.416, "Field Reading"=3.3659143877412356e-09}, {3823.977, "Field Reading"=3.3681157704578086e-09}, {3828.495, "Field Reading"=3.3631301058393767e-09}, {3833.013, "Field Reading"=3.333128492333373e-09}, {3837.54, "Field Reading"=3.3513575047843915e-09}, {3842.102, "Field Reading"=3.366634352724325e-09}, {3846.633, "Field Reading"=3.3800582956665917e-09}, {3851.139, "Field Reading"=3.3549936449744784e-09}, {3855.711, "Field Reading"=3.3350069639059644e-09}, {3860.236, "Field Reading"=3.3547369290268775e-09}, {3864.806, "Field Reading"=3.376196972992089e-09}, {3869.324, "Field Reading"=3.3745771057467733e-09}, {3873.838, "Field Reading"=3.4013985858775113e-09}, {3878.417, "Field Reading"=3.3714903098260553e-09}, {3882.925, "Field Reading"=3.351816746043416e-09}, {3887.442, "Field Reading"=3.343940968194904e-09}, {3892.012, "Field Reading"=3.3320865811731765e-09}, {3896.535, "Field Reading"=3.3570244805781965e-09}, {3901.102, "Field Reading"=3.370095687791086e-09}, {3905.631, "Field Reading"=3.3438506636951637e-09}, {3910.138, "Field Reading"=3.3592381132111537e-09}, {3914.669, "Field Reading"=3.3622020685254113e-09}, {3919.227, "Field Reading"=3.3626764726617746e-09}, {3923.746, "Field Reading"=3.3215220671030723e-09}, {3928.326, "Field Reading"=3.3054788281276907e-09}, {3932.835, "Field Reading"=3.356070787250075e-09}, {3937.352, "Field Reading"=3.34244578169643e-09}, {3941.932, "Field Reading"=3.334460188366267e-09}, {3946.444, "Field Reading"=3.371584609036608e-09}, {3950.961, "Field Reading"=3.3393777531052722e-09}, {3955.54, "Field Reading"=3.3984300323224342e-09}, {3960.055, "Field Reading"=3.3278171859437146e-09}, {3964.618, "Field Reading"=3.3044091545870857e-09}, {3969.137, "Field Reading"=3.3243638363748156e-09}, {3973.655, "Field Reading"=3.330515514248721e-09}, {3978.229, "Field Reading"=3.3154042312525164e-09}, {3982.752, "Field Reading"=3.3325421184594573e-09}, {3987.265, "Field Reading"=3.3073264042472214e-09}, {3991.831, "Field Reading"=3.3242719729558605e-09}, {3996.355, "Field Reading"=3.292889099681115e-09}, {4000.874, "Field Reading"=3.7630882608752615e-09}, {4005.398, "Field Reading"=3.831186949127513e-09}, {4009.957, "Field Reading"=3.799490307245653e-09}, {4014.476, "Field Reading"=3.8197915403744146e-09}, {4019.007, "Field Reading"=3.7912496130880925e-09}, {4023.565, "Field Reading"=3.792913379104307e-09}, {4028.085, "Field Reading"=3.8073529797459035e-09}, {4032.607, "Field Reading"=3.839317592035871e-09}, {4037.174, "Field Reading"=3.7997149156572115e-09}, {4041.691, "Field Reading"=3.800659246430781e-09}, {4046.264, "Field Reading"=3.780545530332075e-09}, {4050.789, "Field Reading"=3.7522129289368205e-09}, {4055.311, "Field Reading"=3.792315687850701e-09}, {4059.871, "Field Reading"=3.777581235143854e-09}, {4064.395, "Field Reading"=3.7495232817596764e-09}, {4068.919, "Field Reading"=3.797812321690146e-09}, {4073.476, "Field Reading"=3.798252377858198e-09}, {4078.003, "Field Reading"=3.8023181576730824e-09}, {4082.564, "Field Reading"=3.806199319361351e-09}, {4087.086, "Field Reading"=3.738555713860219e-09}, {4091.605, "Field Reading"=3.787821611227654e-09}, {4096.131, "Field Reading"=3.754153270702133e-09}, {4100.695, "Field Reading"=3.752343291803743e-09}, {4105.209, "Field Reading"=3.734267664167903e-09}, {4109.734, "Field Reading"=3.753980760293878e-09}, {4114.299, "Field Reading"=3.751732656767793e-09}, {4118.825, "Field Reading"=3.7906412538564455e-09}, {4123.344, "Field Reading"=3.779596504369277e-09}, {4127.909, "Field Reading"=3.775723616309252e-09}, {4132.425, "Field Reading"=3.6930461367211263e-09}, {4136.941, "Field Reading"=3.746284155774599e-09}, {4141.513, "Field Reading"=3.717105633210099e-09}, {4146.031, "Field Reading"=3.734228589421346e-09}, {4150.602, "Field Reading"=3.765009909127514e-09}, {4155.129, "Field Reading"=3.72577062480293e-09}, {4159.637, "Field Reading"=3.754472904525717e-09}, {4164.208, "Field Reading"=3.770048882047128e-09}, {4168.728, "Field Reading"=3.762211629777887e-09}, {4173.244, "Field Reading"=3.732674836804561e-09}, {4177.765, "Field Reading"=3.7456967483633e-09}, {4182.335, "Field Reading"=3.7075462246427387e-09}, {4186.852, "Field Reading"=3.760334785763134e-09}, {4191.421, "Field Reading"=3.823105487655711e-09}, {4195.943, "Field Reading"=3.820723799780019e-09}, {4200.473, "Field Reading"=3.8096294698187016e-09}, {4205.04, "Field Reading"=3.839646220830734e-09}, {4209.559, "Field Reading"=3.814749193475836e-09}, {4214.08, "Field Reading"=3.8415883066738305e-09}, {4218.637, "Field Reading"=3.870896087610181e-09}, {4223.164, "Field Reading"=3.84339915009081e-09}, {4227.731, "Field Reading"=3.855657427412204e-09}, {4232.244, "Field Reading"=3.83758649018947e-09}, {4236.773, "Field Reading"=3.780015605512126e-09}, {4241.339, "Field Reading"=3.781684653602896e-09}, {4245.849, "Field Reading"=3.804079773485682e-09}, {4250.38, "Field Reading"=3.812682173556427e-09}, {4254.941, "Field Reading"=3.780886428472993e-09}, {4259.459, "Field Reading"=3.813844745667443e-09}, {4264.027, "Field Reading"=3.808062998558914e-09}, {4268.556, "Field Reading"=3.778519845202089e-09}, {4273.068, "Field Reading"=3.795867584151631e-09}, {4277.584, "Field Reading"=3.781566609661007e-09}, {4282.155, "Field Reading"=3.876786945839434e-09}, {4286.682, "Field Reading"=3.783566925216681e-09}, {4291.243, "Field Reading"=3.820081077551572e-09}, {4295.771, "Field Reading"=3.78379020933242e-09}, {4300.281, "Field Reading"=3.662766013240078e-09}, {4304.857, "Field Reading"=3.692840758214636e-09}, {4309.368, "Field Reading"=3.730041385881614e-09}, {4313.885, "Field Reading"=3.7062392675322523e-09}, {4318.408, "Field Reading"=3.654104985820504e-09}, {4322.975, "Field Reading"=3.6402148541522486e-09}, {4327.492, "Field Reading"=3.7011219149946424e-09}, {4332.074, "Field Reading"=3.653562552792899e-09}, {4336.581, "Field Reading"=3.749450403239406e-09}, {4341.113, "Field Reading"=3.698835478243219e-09}, {4345.673, "Field Reading"=3.7210017416001658e-09}, {4350.202, "Field Reading"=3.678323807294075e-09}, {4354.711, "Field Reading"=3.6792994057081684e-09}, {4359.279, "Field Reading"=3.664190406810518e-09}, {4363.8, "Field Reading"=3.6478108460634436e-09}, {4368.365, "Field Reading"=3.6822893005096643e-09}, {4372.894, "Field Reading"=3.6858896516747643e-09}, {4377.405, "Field Reading"=3.707543536333386e-09}, {4381.926, "Field Reading"=3.6590095703143432e-09}, {4386.493, "Field Reading"=3.6931662977642644e-09}, {4391.023, "Field Reading"=3.6770874204482614e-09}, {4395.58, "Field Reading"=3.6887459128446484e-09}, {4400.11, "Field Reading"=3.635805127286088e-09}, {4404.625, "Field Reading"=3.670779152379082e-09}, {4409.14, "Field Reading"=3.660554121018082e-09}, {4413.718, "Field Reading"=3.722231111970162e-09}, {4418.229, "Field Reading"=3.642575974878886e-09}, {4422.796, "Field Reading"=3.639067261461371e-09}, {4427.317, "Field Reading"=3.6533612643531043e-09}, {4431.843, "Field Reading"=3.727511443781943e-09}, {4436.402, "Field Reading"=3.6555019886780653e-09}, {4440.928, "Field Reading"=3.6500288269725488e-09}, {4445.45, "Field Reading"=3.674086075675457e-09}, {4450.021, "Field Reading"=3.620086550149377e-09}, {4454.539, "Field Reading"=3.660094603182133e-09}, {4459.047, "Field Reading"=3.682457257366845e-09}, {4463.629, "Field Reading"=3.686580732752353e-09}, {4468.138, "Field Reading"=3.6823260190164972e-09}, {4472.667, "Field Reading"=3.655396638110982e-09}, {4477.226, "Field Reading"=3.648021953416541e-09}, {4481.745, "Field Reading"=3.617186137484899e-09}, {4486.273, "Field Reading"=3.700816873758431e-09}, {4490.831, "Field Reading"=3.6475672047889485e-09}, {4495.361, "Field Reading"=3.6446538765545973e-09}, {4499.871, "Field Reading"=3.6445156548201866e-09}, {4504.448, "Field Reading"=3.6545776613728108e-09}, {4508.96, "Field Reading"=3.6418264958176964e-09}, {4513.48, "Field Reading"=3.6118585280536836e-09}, {4518.044, "Field Reading"=3.627462141311246e-09}, {4522.578, "Field Reading"=3.6509622236937597e-09}, {4527.084, "Field Reading"=3.614311999060243e-09}, {4531.666, "Field Reading"=3.6077779160949212e-09}, {4536.174, "Field Reading"=3.587597204518528e-09}, {4540.745, "Field Reading"=3.637945219050798e-09}, {4545.266, "Field Reading"=3.6661029812026346e-09}, {4549.782, "Field Reading"=3.573393224241141e-09}, {4554.299, "Field Reading"=3.612175862252782e-09}, {4558.877, "Field Reading"=3.615067535138304e-09}, {4563.398, "Field Reading"=3.614671181220314e-09}, {4567.954, "Field Reading"=3.6500174692117803e-09}, {4572.476, "Field Reading"=3.6290960651785084e-09}, {4576.992, "Field Reading"=3.6015553711966363e-09}, {4581.515, "Field Reading"=3.573684719957642e-09}, {4586.082, "Field Reading"=3.5945241828636324e-09}, {4590.607, "Field Reading"=3.5890667563632073e-09}, {4595.129, "Field Reading"=3.609937661134198e-09}, {4599.699, "Field Reading"=3.588611418372969e-09}, {4604.21, "Field Reading"=3.593696304503749e-09}, {4608.781, "Field Reading"=3.6296754760254136e-09}, {4613.298, "Field Reading"=3.5977236250261366e-09}, {4617.826, "Field Reading"=3.5577064971055857e-09}, {4622.387, "Field Reading"=3.5968320628404765e-09}, {4626.907, "Field Reading"=3.5834847245089322e-09}, {4631.434, "Field Reading"=3.6215126771494063e-09}, {4635.992, "Field Reading"=3.5341010780107447e-09}, {4640.522, "Field Reading"=3.6145604517956024e-09}, {4645.043, "Field Reading"=3.5610127883629683e-09}, {4649.598, "Field Reading"=3.5811078967803045e-09}, {4654.119, "Field Reading"=3.5673237567194094e-09}, {4658.645, "Field Reading"=3.5678133864067906e-09}, {4663.207, "Field Reading"=3.6585745606224573e-09}, {4667.727, "Field Reading"=3.619673934526269e-09}, {4672.296, "Field Reading"=3.6073350300460914e-09}, {4676.816, "Field Reading"=3.6327616168727266e-09}, {4681.333, "Field Reading"=3.558136662411252e-09}, {4685.854, "Field Reading"=3.570447387946343e-09}, {4690.422, "Field Reading"=3.5539304830551027e-09}, {4694.95, "Field Reading"=3.5353241968053985e-09}, {4699.523, "Field Reading"=3.5506358584504986e-09}, {4704.032, "Field Reading"=3.6414144417691487e-09}, {4708.548, "Field Reading"=3.549243397164856e-09}, {4713.131, "Field Reading"=3.5919030403772616e-09}, {4717.647, "Field Reading"=3.6014146244012975e-09}, {4722.154, "Field Reading"=3.5743151620009123e-09}, {4726.726, "Field Reading"=3.564590097655378e-09}, {4731.251, "Field Reading"=3.5874397834560595e-09}, {4735.776, "Field Reading"=3.5760230268114953e-09}, {4740.334, "Field Reading"=3.576704109068708e-09}, {4744.853, "Field Reading"=3.5803029624922167e-09}, {4749.369, "Field Reading"=3.546618860181526e-09}, {4753.948, "Field Reading"=3.5637739327551106e-09}, {4758.459, "Field Reading"=3.5567617353012513e-09}, {4763.03, "Field Reading"=3.564906764731017e-09}, {4767.554, "Field Reading"=3.591471707235843e-09}, {4772.073, "Field Reading"=3.574682407759251e-09}, {4776.636, "Field Reading"=3.5290719552360317e-09}, {4781.153, "Field Reading"=3.533263874164214e-09}, {4785.684, "Field Reading"=3.5742186594946835e-09}, {4790.255, "Field Reading"=3.569169605670257e-09}, {4794.761, "Field Reading"=3.563017205963788e-09}, {4799.28, "Field Reading"=3.63989107652287e-09}, {4803.858, "Field Reading"=3.5921670708105104e-09}, {4808.378, "Field Reading"=3.5907813725965584e-09}, {4812.893, "Field Reading"=3.5685972435327887e-09}, {4817.459, "Field Reading"=3.414508950847085e-09}, {4821.988, "Field Reading"=3.528404975216492e-09}, {4826.494, "Field Reading"=3.543126041045317e-09}, {4831.071, "Field Reading"=3.5022041837728537e-09}, {4835.592, "Field Reading"=3.5615907383049575e-09}, {4840.161, "Field Reading"=3.5485356729084723e-09}, {4844.629, "Field Reading"=3.5423158111164783e-09}, {4849.202, "Field Reading"=3.5434547202933622e-09}, {4853.708, "Field Reading"=3.567843449160732e-09}, {4858.287, "Field Reading"=3.5606686698245152e-09}, {4862.798, "Field Reading"=3.53066942237924e-09}, {4867.319, "Field Reading"=3.5505758077643977e-09}, {4871.898, "Field Reading"=3.538233085857631e-09}, {4876.406, "Field Reading"=3.532006910514881e-09}, {4880.932, "Field Reading"=3.5560910769982047e-09}, {4885.501, "Field Reading"=3.524835165122796e-09}, {4890.011, "Field Reading"=3.52452294668333e-09}, {4894.539, "Field Reading"=3.5357207673635034e-09}, {4899.103, "Field Reading"=3.5076157566867513e-09}, {4903.622, "Field Reading"=3.5679838633043687e-09}, {4908.142, "Field Reading"=3.5282113347638255e-09}, {4912.716, "Field Reading"=3.5147989339135775e-09}, {4917.228, "Field Reading"=3.5129506262271114e-09}, {4921.745, "Field Reading"=3.535850638324042e-09}, {4926.315, "Field Reading"=3.5304725205838635e-09}, {4930.847, "Field Reading"=3.5125103352639776e-09}, {4935.355, "Field Reading"=3.5340281893501223e-09}, {4939.923, "Field Reading"=3.5254658575470236e-09}, {4944.453, "Field Reading"=3.4658812735369297e-09}, {4949.021, "Field Reading"=3.538557568632987e-09}, {4953.53, "Field Reading"=3.536894766831468e-09}, {4958.051, "Field Reading"=3.5052771181927623e-09}, {4962.57, "Field Reading"=3.4908767640122804e-09}, {4967.147, "Field Reading"=3.5128966153982362e-09}, {4971.666, "Field Reading"=3.4965604256913124e-09}, {4976.178, "Field Reading"=3.508436337590528e-09}, {4980.746, "Field Reading"=3.518893010981431e-09}, {4985.264, "Field Reading"=3.5108602046628896e-09}, {4989.84, "Field Reading"=3.508034600903703e-09}, {4994.361, "Field Reading"=3.526566969332725e-09}, {4998.87, "Field Reading"=3.5290707450303005e-09}, {5003.393, "Field Reading"=3.5247825627216746e-09}, {5007.961, "Field Reading"=3.5155625558238e-09}, {5012.493, "Field Reading"=3.4832808180225957e-09}, {5017.059, "Field Reading"=3.4631802684256766e-09}, {5021.577, "Field Reading"=3.5245382279830744e-09}, {5026.087, "Field Reading"=3.493014503661058e-09}, {5030.664, "Field Reading"=3.5077440603638933e-09}, {5035.181, "Field Reading"=3.516808482188399e-09}, {5039.696, "Field Reading"=3.512097439822284e-09}, {5044.26, "Field Reading"=3.507970387115964e-09}, {5048.789, "Field Reading"=3.5441436944002487e-09}, {5053.298, "Field Reading"=3.5472454205405112e-09}, {5057.874, "Field Reading"=3.515938234586467e-09}, {5062.398, "Field Reading"=3.5114183637472307e-09}, {5066.913, "Field Reading"=3.5131105697440206e-09}, {5071.478, "Field Reading"=3.489409925233194e-09}, {5075.996, "Field Reading"=3.5412122106542376e-09}, {5080.563, "Field Reading"=3.4889555330674893e-09}, {5085.085, "Field Reading"=3.5554900261421475e-09}, {5089.655, "Field Reading"=3.5431862505908345e-09}, {5094.175, "Field Reading"=3.5585538487205798e-09}, {5098.702, "Field Reading"=3.5421208257378886e-09}, {5103.212, "Field Reading"=3.5641157183364437e-09}, {5107.78, "Field Reading"=3.4965062651483517e-09}, {5112.307, "Field Reading"=3.559852107419659e-09}, {5116.87, "Field Reading"=3.573927004340061e-09}, {5121.383, "Field Reading"=3.5318300404194132e-09}, {5125.904, "Field Reading"=3.5440284969451353e-09}, {5130.425, "Field Reading"=3.5269449106798734e-09}, {5134.994, "Field Reading"=3.5419765181973824e-09}, {5139.516, "Field Reading"=3.5630802647693873e-09}, {5144.028, "Field Reading"=3.5584962136368724e-09}, {5148.551, "Field Reading"=3.5285613278590076e-09}, {5153.129, "Field Reading"=3.525299151482247e-09}, {5157.639, "Field Reading"=3.5248076297893948e-09}, {5162.208, "Field Reading"=3.4993755307357826e-09}, {5166.737, "Field Reading"=3.4980396500871575e-09}, {5171.293, "Field Reading"=3.522935689421467e-09}, {5175.819, "Field Reading"=3.542807999715702e-09}, {5180.341, "Field Reading"=3.5231335245865022e-09}, {5184.906, "Field Reading"=3.5608667997570613e-09}, {5189.426, "Field Reading"=3.3848774550661942e-09}, {5193.952, "Field Reading"=3.527467303547001e-09}, {5198.514, "Field Reading"=3.490919244342005e-09}, {5203.031, "Field Reading"=3.5255564254727164e-09}, {5207.558, "Field Reading"=3.5716786500674394e-09}, {5212.12, "Field Reading"=3.6616602154730677e-09}, {5216.642, "Field Reading"=3.532684091414905e-09}, {5221.156, "Field Reading"=3.5084430666921276e-09}, {5225.734, "Field Reading"=3.5107743221246077e-09}, {5230.253, "Field Reading"=3.514647995387958e-09}, {5234.773, "Field Reading"=3.4714694183279203e-09}, {5239.339, "Field Reading"=3.5081045757948136e-09}, {5243.853, "Field Reading"=3.5133156703924012e-09}, {5248.431, "Field Reading"=3.513959546355283e-09}, {5252.941, "Field Reading"=3.522213566477419e-09}, {5257.459, "Field Reading"=3.5100062690402514e-09}, {5262.029, "Field Reading"=3.568948049730121e-09}, {5266.547, "Field Reading"=3.5035845358938084e-09}, {5271.065, "Field Reading"=3.5959552427106783e-09}, {5275.585, "Field Reading"=3.471282575660944e-09}, {5280.165, "Field Reading"=3.505981295098846e-09}, {5284.676, "Field Reading"=3.5035137454019685e-09}, {5289.201, "Field Reading"=3.5325421587968997e-09}, {5293.722, "Field Reading"=3.507649773327779e-09}, {5298.287, "Field Reading"=3.5125470922041546e-09}, {5302.814, "Field Reading"=3.4723036383845107e-09}, {5307.367, "Field Reading"=3.5174281005628937e-09}, {5311.887, "Field Reading"=3.4883174300600597e-09}, {5316.408, "Field Reading"=3.5213262917658748e-09}, {5320.978, "Field Reading"=3.506188505241338e-09}, {5325.497, "Field Reading"=3.5121075818672438e-09}, {5330.037, "Field Reading"=3.510021325672779e-09}, {5334.588, "Field Reading"=3.4879177669245874e-09}, {5339.116, "Field Reading"=3.4944205127865978e-09}, {5343.62, "Field Reading"=3.467162649439533e-09}, {5348.192, "Field Reading"=3.4974912813007444e-09}, {5352.713, "Field Reading"=3.4713003591186177e-09}, {5357.233, "Field Reading"=3.5119563395917646e-09}, {5361.807, "Field Reading"=3.478622864956187e-09}, {5366.326, "Field Reading"=3.518182476058491e-09}, {5370.894, "Field Reading"=3.5161496946581007e-09}, {5375.408, "Field Reading"=3.484072436808271e-09}, {5379.931, "Field Reading"=3.5218858630250192e-09}, {5384.494, "Field Reading"=3.5278473495616228e-09}, {5389.014, "Field Reading"=3.385519606009418e-09}, {5393.542, "Field Reading"=3.529878574143357e-09}, {5398.1, "Field Reading"=3.5129372170889224e-09}, {5402.623, "Field Reading"=3.5293187474612565e-09}, {5407.137, "Field Reading"=3.5310430427565642e-09}, {5411.712, "Field Reading"=3.5186123563782437e-09}, {5416.239, "Field Reading"=3.5500484860969204e-09}, {5420.745, "Field Reading"=3.5186788267384596e-09}, {5425.266, "Field Reading"=3.5684715702220438e-09}, {5429.833, "Field Reading"=3.5588909586491285e-09}, {5434.353, "Field Reading"=3.5388618023993446e-09}, {5438.923, "Field Reading"=3.5585328785296407e-09}, {5443.452, "Field Reading"=3.466137039866585e-09}, {5447.962, "Field Reading"=3.5130940202296452e-09}, {5452.53, "Field Reading"=3.5042936027454083e-09}, {5457.058, "Field Reading"=3.533541295807816e-09}, {5461.628, "Field Reading"=3.5448439921311412e-09}, {5466.136, "Field Reading"=3.5688545116011245e-09}, {5470.657, "Field Reading"=3.555733346240926e-09}, {5475.175, "Field Reading"=3.5386387673765522e-09}, {5479.747, "Field Reading"=3.5258869695074785e-09}, {5484.267, "Field Reading"=3.515057065544191e-09}, {5488.835, "Field Reading"=3.495183518416594e-09}, {5493.353, "Field Reading"=3.5037794560346154e-09}, {5497.882, "Field Reading"=3.5047651126837122e-09}, {5502.455, "Field Reading"=3.527159577345344e-09}, {5506.967, "Field Reading"=3.518258167127279e-09}, {5511.483, "Field Reading"=3.5336599355919646e-09}, {5516.05, "Field Reading"=3.5243804918642543e-09}, {5520.569, "Field Reading"=3.514576169199349e-09}, {5525.086, "Field Reading"=3.512209995516481e-09}, {5529.664, "Field Reading"=3.5192045573477372e-09}, {5534.18, "Field Reading"=3.520247209976684e-09}, {5538.744, "Field Reading"=3.4246995089583774e-09}, {5543.263, "Field Reading"=3.417000948008042e-09}, {5547.783, "Field Reading"=3.410679517033019e-09}, {5552.35, "Field Reading"=3.4205524970295896e-09}, {5556.879, "Field Reading"=3.4070714574897358e-09}, {5561.392, "Field Reading"=3.4135738331336225e-09}, {5565.96, "Field Reading"=3.4228074907860684e-09}, {5570.479, "Field Reading"=3.411922153539338e-09}, {5575.006, "Field Reading"=3.429626615102948e-09}, {5579.522, "Field Reading"=3.397491063831622e-09}, {5584.099, "Field Reading"=3.3602365174304575e-09}, {5588.603, "Field Reading"=3.410935443199188e-09}, {5593.181, "Field Reading"=3.3804768191344434e-09}, {5597.694, "Field Reading"=3.366305273426794e-09}, {5602.217, "Field Reading"=3.4124408247864353e-09}, {5606.788, "Field Reading"=3.3520954107723816e-09}, {5611.299, "Field Reading"=3.3702111786258594e-09}, {5615.826, "Field Reading"=3.640788358243646e-09}, {5620.391, "Field Reading"=3.6339887892004364e-09}, {5624.907, "Field Reading"=3.6591467890772594e-09}, {5629.426, "Field Reading"=3.654337596478476e-09}, {5633.994, "Field Reading"=3.4344425035816366e-09}, {5638.512, "Field Reading"=3.3197226018076897e-09}, {5643.035, "Field Reading"=3.3316909524986355e-09}, {5647.601, "Field Reading"=3.359643422359665e-09}, {5652.119, "Field Reading"=3.3248047534887974e-09}, {5656.693, "Field Reading"=3.3178754339417863e-09}, {5661.209, "Field Reading"=3.3115923471097545e-09}, {5665.731, "Field Reading"=3.3470520798677666e-09}, {5670.298, "Field Reading"=3.2986486295232833e-09}, {5674.827, "Field Reading"=3.3347739836301624e-09}, {5679.341, "Field Reading"=3.3783963636163155e-09}, {5683.905, "Field Reading"=3.3190741852539347e-09}, {5688.435, "Field Reading"=3.344870356515067e-09}, {5693.004, "Field Reading"=3.2915535775259492e-09}, {5697.524, "Field Reading"=3.3698026925649132e-09}, {5702.042, "Field Reading"=3.2913075494416435e-09}, {5706.608, "Field Reading"=3.364075537758397e-09}, {5711.12, "Field Reading"=3.378381001440542e-09}, {5715.642, "Field Reading"=3.338440219929952e-09}, {5720.206, "Field Reading"=3.370006130768135e-09}, {5724.736, "Field Reading"=3.348953846635677e-09}, {5729.243, "Field Reading"=3.393314107634969e-09}, {5733.817, "Field Reading"=3.36826357572448e-09}, {5738.34, "Field Reading"=3.4044755953995495e-09}, {5742.86, "Field Reading"=3.294084379308686e-09}, {5747.373, "Field Reading"=3.3064460244823006e-09}, {5751.95, "Field Reading"=3.282439032671958e-09}, {5756.47, "Field Reading"=3.352030922746977e-09}, {5761.029, "Field Reading"=3.3001370876834917e-09}, {5765.556, "Field Reading"=3.2861463084600455e-09}, {5770.074, "Field Reading"=3.2939605602096916e-09}, {5774.637, "Field Reading"=3.311076553270725e-09}, {5779.154, "Field Reading"=3.3248621663939657e-09}, {5783.685, "Field Reading"=3.295155433999231e-09}, {5788.202, "Field Reading"=3.2557371111642765e-09}, {5792.773, "Field Reading"=3.294171543032423e-09}, {5797.28, "Field Reading"=3.303481870196785e-09}, {5801.848, "Field Reading"=3.281545361638774e-09}, {5806.38, "Field Reading"=3.3121328043901257e-09}, {5810.9, "Field Reading"=3.3865210102615373e-09}, {5815.466, "Field Reading"=3.412564785189739e-09}, {5819.974, "Field Reading"=3.42770492453106e-09}, {5824.51, "Field Reading"=3.402680031328693e-09}, {5829.013, "Field Reading"=3.429255265304855e-09}, {5833.588, "Field Reading"=3.4205888225075647e-09}, {5838.103, "Field Reading"=3.4073593291641222e-09}, {5842.625, "Field Reading"=3.4472893219236477e-09}, {5847.19, "Field Reading"=3.405920252493065e-09}, {5851.72, "Field Reading"=3.4011559367406734e-09}, {5856.228, "Field Reading"=3.3937431684717476e-09}, {5860.808, "Field Reading"=3.3960953688060427e-09}, {5865.327, "Field Reading"=3.4039249278822036e-09}, {5869.849, "Field Reading"=3.3805622476033857e-09}, {5874.415, "Field Reading"=3.38616405994008e-09}, {5878.924, "Field Reading"=3.417640789250558e-09}, {5883.443, "Field Reading"=3.4037277625568886e-09}, {5888.014, "Field Reading"=3.3582995742366617e-09}, {5892.533, "Field Reading"=3.397176106996993e-09}, {5897.104, "Field Reading"=3.4085880693043634e-09}, {5901.623, "Field Reading"=3.4052831452819543e-09}, {5906.148, "Field Reading"=3.361169937525962e-09}, {5910.658, "Field Reading"=3.3772097793542677e-09}, {5915.238, "Field Reading"=3.4021137207509774e-09}, {5919.756, "Field Reading"=3.381986029529632e-09}, {5924.333, "Field Reading"=3.3719548944924975e-09}]
  in  "?":bool
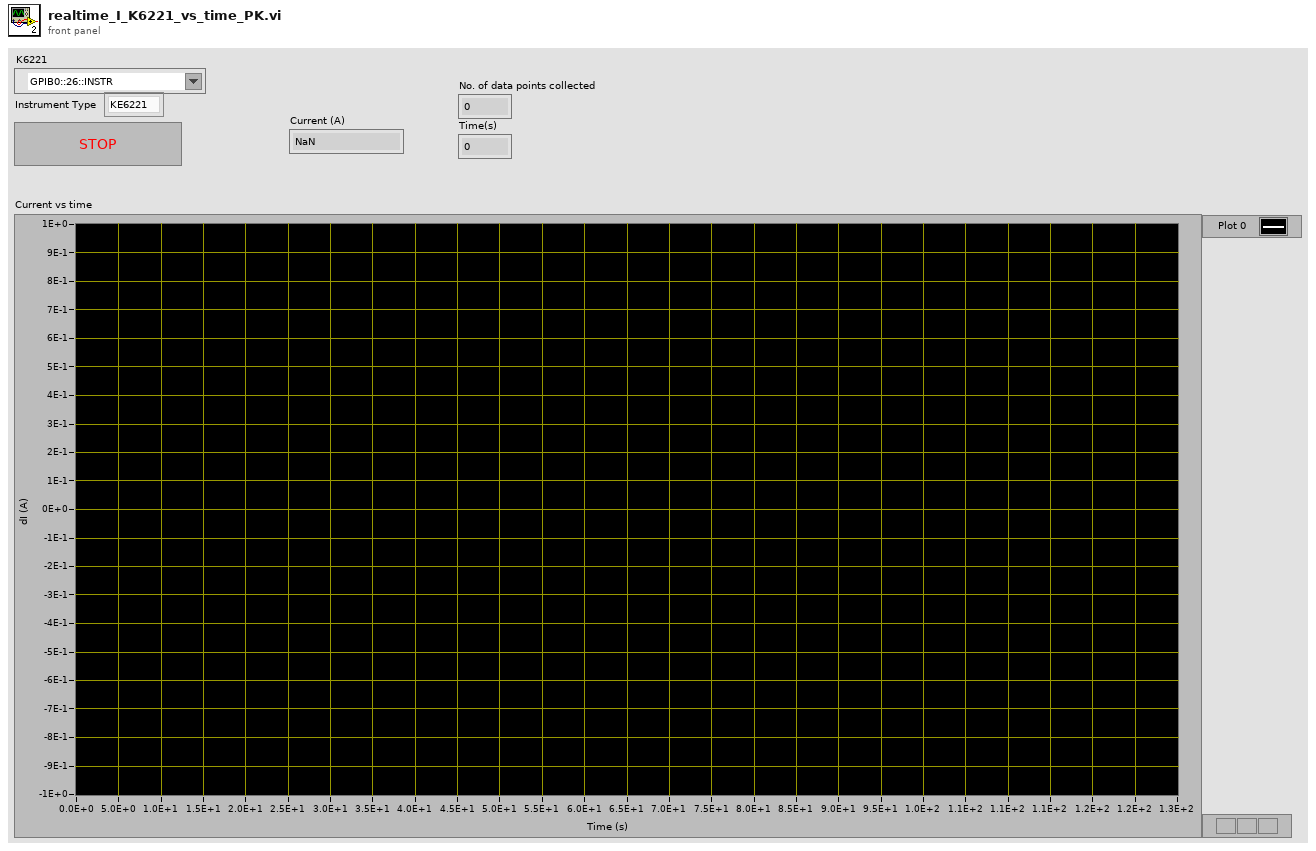
[diagram p1: front panel]
types:
  T1 = typedef "Keithley 622x.lvlib/KE622x -- Instrument Type.ctl" = enum16{"KE6220", "KE6221"}
  T2 = typedef "Keithley 622x.lvlib/KE622x -- Current Level.ctl" = dbl
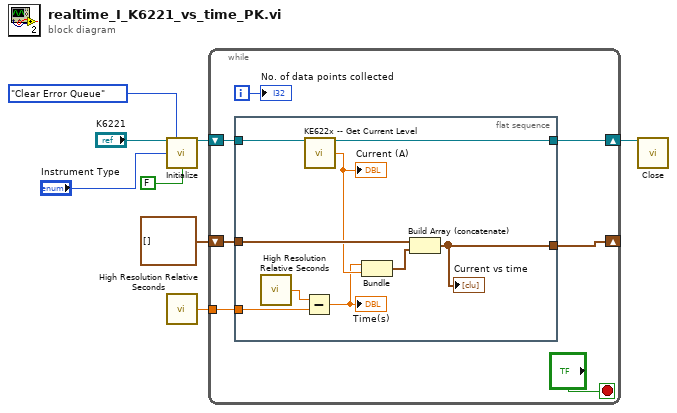
[diagram p0: block diagram]
diagram:
  n1 = call <instrlib>:"Initialize.vi"("VISA resource name"="K6221", "Error Queue Option"=enum16{"Clear Error Queue", "Error Query"}."Clear Error Queue", "Instrument Type"="Instrument Type", "Reset? (T)"=FALSE) -> ("VISA resource name out"=w5:refnum<visa-resource-name>)  [unwired: 10 in, 1 out]
  n2 = call <vilib>:"High Resolution Relative Seconds.vi"() -> ("relative seconds"=w4:dbl)
  n3 = while {
    tunnel: w4 -> [w15]
    shift-right: [w12] -> _
    shift-left: cluster{dbl, "Field Reading":dbl}[] [] -> [w13]
    shift-right: [w9] -> w3
    shift-left: w5 -> [w10]
    i -> [w11]
    stop <- "?" stop-if-true
    n4 = flat-sequence {
      tunnel: w13 -> [w22]
      tunnel: [w21] -> w12
      tunnel: w15 -> [w24]
      tunnel: w10 -> [w19]
      tunnel: [w17] -> w9
      frame #0 {
        n5 = call <vilib>:"High Resolution Relative Seconds.vi"() -> ("relative seconds"=w18:dbl)
        n6 = Subtract(x=w18, y=w24) -> (x-y=w16:dbl)
        "Time(s)" <- w16
        n7 = call <instrlib>:"KE622x -- Get Current Level.vi"("Resource In"=w19) -> ("Resource Out (dupl)"=w17:refnum<visa-resource-name>, "Current Level (A)"=w20:T2)  [unwired: 12 in, 1 out]
        "Current (A)" <- w20
        n8 = Bundle(w16, "Current Level (A)"=w20) -> (w23:cluster{dbl, "Current Level (A)":T2})  [unwired: 1 in]
        n9 = Build Array (concatenate)(w22, w23) -> (w21:cluster{dbl, "Current Level (A)":T2}[])
        "Current vs time" <- w21
      }
    }
    "No. of data points collected" <- w11
  }
  n10 = call <instrlib>:"Close.vi"("VISA resource name"=w3) -> ()  [unwired: 14 in, 1 out]
